vi "main.vi"() -> ()   [LabVIEW 2020]
uses:
  Newport.XPS.CommandInterface
panel:
  out "GatheringStopAndSave":i32
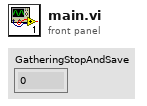
[diagram p1: front panel]
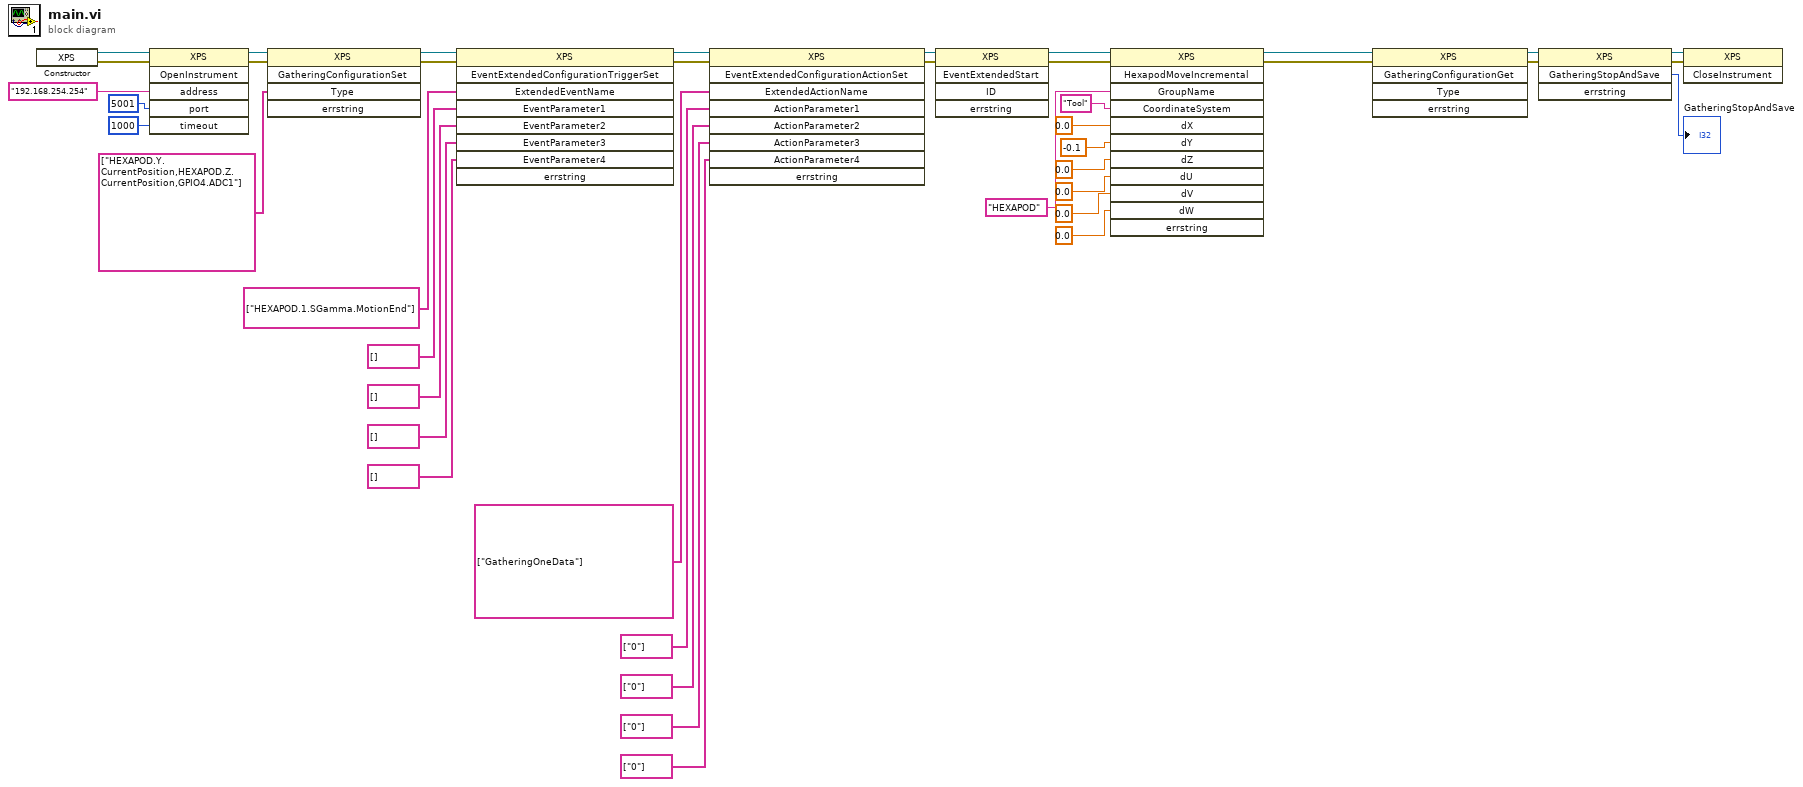
[diagram p0: block diagram]
diagram:
  n1 = constructor class="XPS"() -> (reference out=w16:refnum<k24>, error out=w15:errorcluster)  [unwired: 3 in, 1 out]
  n2 = invoke on="Nœud de méthode" class="XPS" method="OpenInstrument"(reference=w16, error in=w15, "address"="192.168.254.254", "port"=5001, "timeout"=1000) -> (reference out=w26:refnum<k24>, error out=w25:errorcluster)  [unwired: 1 in, 4 out]
  n3 = invoke on="Nœud de méthode" class="XPS" method="GatheringConfigurationSet"(reference=w26, error in=w25, "Type"=string[] ["HEXAPOD.Y.CurrentPosition,HEXAPOD.Z.CurrentPosition,GPIO4.ADC1"]) -> (reference out=w24:refnum<k24>, error out=w23:errorcluster)  [unwired: 2 in, 3 out]
  n4 = invoke on="Nœud de méthode" class="XPS" method="EventExtendedConfigurationTriggerSet"(reference=w24, error in=w23, "ExtendedEventName"=string[] ["HEXAPOD.1.SGamma.MotionEnd"], "EventParameter1"=string[] [], "EventParameter2"=string[] [], "EventParameter3"=string[] [], "EventParameter4"=string[] []) -> (reference out=w22:refnum<k24>, error out=w21:errorcluster)  [unwired: 2 in, 7 out]
  n5 = invoke on="Nœud de méthode" class="XPS" method="EventExtendedConfigurationActionSet"(reference=w22, error in=w21, "ExtendedActionName"=string[] ["GatheringOneData"], "ActionParameter1"=string[] ["0"], "ActionParameter2"=string[] ["0"], "ActionParameter3"=string[] ["0"], "ActionParameter4"=string[] ["0"]) -> (reference out=w20:refnum<k24>, error out=w19:errorcluster)  [unwired: 2 in, 7 out]
  n6 = invoke on="Nœud de méthode" class="XPS" method="EventExtendedStart"(reference=w20, error in=w19) -> (reference out=w6:refnum<k24>, error out=w5:errorcluster)  [unwired: 3 in, 3 out]
  n7 = invoke on="Nœud de méthode" class="XPS" method="HexapodMoveIncremental"(reference=w6, error in=w5, "GroupName"="HEXAPOD", "CoordinateSystem"="Tool", "dX"=0.0, "dY"=-0.1, "dZ"=0.0, "dU"=0.0, "dV"=0.0, "dW"=0.0) -> (reference out=w4:refnum<k24>, error out=w3:errorcluster)  [unwired: 2 in, 10 out]
  n8 = invoke on="Nœud de méthode" class="XPS" method="GatheringConfigurationGet"(reference=w4, error in=w3) -> (reference out=w2:refnum<k24>, error out=w1:errorcluster)  [unwired: 3 in, 3 out]
  n9 = invoke on="Nœud de méthode" class="XPS" method="GatheringStopAndSave"(reference=w2, error in=w1) -> (reference out=w17:refnum<k24>, error out=w18:errorcluster, "GatheringStopAndSave"=→"GatheringStopAndSave":i32)  [unwired: 2 in, 1 out]
  n10 = invoke on="Nœud de méthode" class="XPS" method="CloseInstrument"(reference=w17, error in=w18) -> ()  [unwired: 1 in, 3 out]
